vi "SetParam.vi"(8 "error in (no error)":errorcluster caption="entrée d'erreur (pas d'erreur)", 10 "make_moons":T1={"n_samples"="100", "shuffle"=TRUE, "noise"=-1.0, "random_state"=-1, "Returns"="X"} {"noise" min=-1.0; "random_state" min=-1}, 11 "Moons.lvclass":refnum<class "Moons.lvclass">) -> (0 "error out":errorcluster caption="sortie d'erreur", 3 "Moons.lvclass":refnum<class "Moons.lvclass">)   [LabVIEW 2020, in "Moons.lvclass"]
doc: "Set Parameters"
uses:
  Moons.lvclass
  Moons.lvclass/Moons.ctl
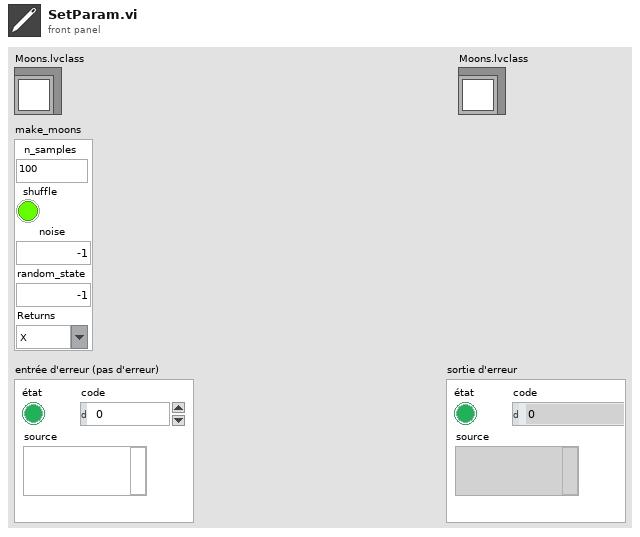
[diagram p1: front panel]
types:
  T1 = cluster{"n_samples":string, "shuffle":bool, "noise":dbl, "random_state":i32, "Returns":string}
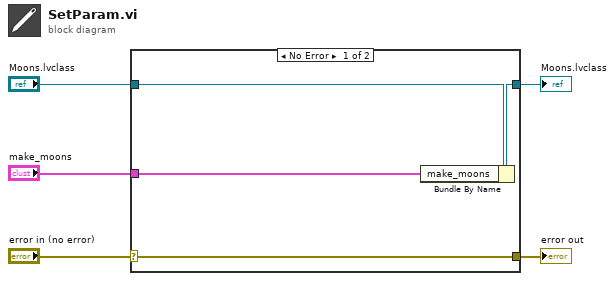
[diagram p0: block diagram]
diagram:
  n1 = case shown="No Error" "error in (no error)" {
    selector: "error in (no error)" -> [w9 w10]
    tunnel: [w9 w10] -> w4
    tunnel: [w7 w11] -> w2
    tunnel: "Moons.lvclass" -> [w8 w11]
    tunnel: "make_moons" -> [w6 _]
    frame No Error {
      n2 = Bundle By Name(cluster=w8, "make_moons"=w6) -> (w7:refnum<class "Moons.lvclass">)
    }
    frame Error {
    }
  }
  "error out" <- w4
  "Moons.lvclass" <- w2
